vi "Build Hierarchy Map.vi"(9 "Hierarchies":cluster{"Hierarchy":string[]}[](array[cluster]), 10 "Elements in":refnum<class "Config Element.lvclass">[](array[class])) -> (1 "Children Map":map{string[], set{string[]}}(c390), 2 "Name Map":T1(c390))   [LabVIEW 2020, in "CDM-Config.lvlib" / "Config Manager.lvclass"]
uses:
  Config Manager.lvclass
  Config Manager.lvclass/Config Manager.ctl
  <vilib>/Utility/miscctls.llb/LVMapReplaceAction.ctl
  Config Element/Config Element.lvclass
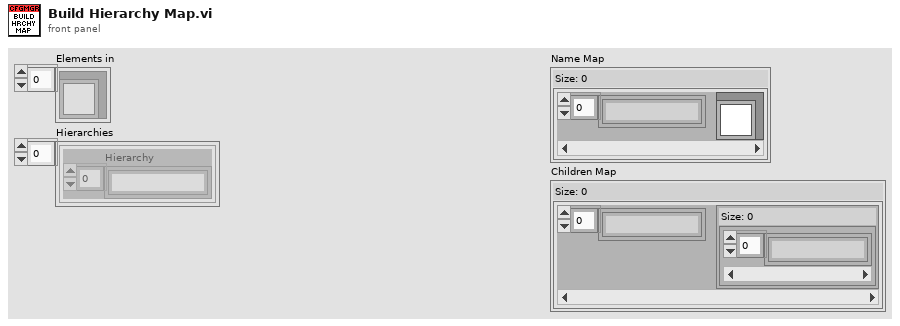
[diagram p1: front panel]
types:
  T1 = map{string[], refnum<class "Config Element.lvclass">}
  T2 = typedef "LVMapReplaceAction.ctl" = enum32{"Modify Entry only if found", "Add or Modify Entry", "Delete Entry"}
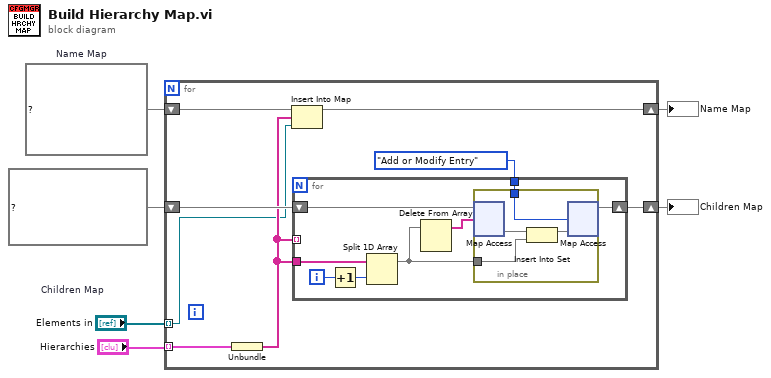
[diagram p0: block diagram]
diagram:
  w5 = T1 {}  # Name Map
  w6 = map{string[], set{string[]}} {}  # Children Map
  n1 = for {
    tunnel: "Elements in" -> [w7] mode=indexing
    shift-right: [w11] -> w1
    shift-left: w6 -> [w14]
    shift-right: [w12] -> w2
    shift-left: w5 -> [w13]
    tunnel: "Hierarchies" -> [w9] mode=indexing
    n2 = Unbundle(w9) -> ("Hierarchy"=w8:string[])
    n3 = Insert Into Map(map in=w13, key=w8, value=w7) -> (map out=w12:T1)  [unwired: 2 out]
    n4 = for {
      shift-right: [w21] -> w11
      shift-left: w14 -> [w22]
      tunnel: w8 -> [w18]
      tunnel: LVMapReplaceAction."Add or Modify Entry" ("action") -> [w15]
      tunnel: w8 -> [_] mode=indexing
      i -> [w20]
      n5 = Increment(x=w20) -> (x+1=w19:i32)
      n6 = Split 1D Array(array=w18, index=w19) -> (first subarray=w16:string[])  [unwired: 1 out]
      n7 = Delete From Array(array=w16) -> (array with subset deleted=w17:string[])  [unwired: 2 in, 1 out]
      n8 = in-place {
        in-place-border: w16 -> [w24]
        in-place-border: w15 -> [w23]
        n9 = in-place-map #1(w22, w17) -> (w26:set{string[]})  [unwired: 1 in, 1 out]
        n10 = Insert Into Set(10:w24, 11:w26) -> (3:w25:set{string[]})  [unwired: 1 out]
        n11 = in-place-map #1(w25, w23) -> (w21:map{string[], set{string[]}})  [unwired: 2 out]
      }
    }
  }
  "Name Map" <- w2
  "Children Map" <- w1
